vi "Cleanup Session.vi"(8 "error in":errorcluster, 11 "Plugin in":refnum<class "Output Sequencer.lvclass">) -> (0 "error out":errorcluster, 3 "Plugin out":refnum<class "Output Sequencer.lvclass">)   [LabVIEW 2024, in "Output Sequencer.lvlib" / "Output Sequencer.lvclass"]
uses:
  Output Sequencer.lvclass
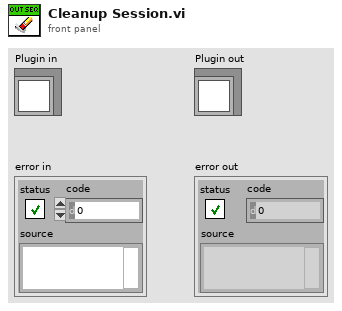
[diagram p1: front panel]
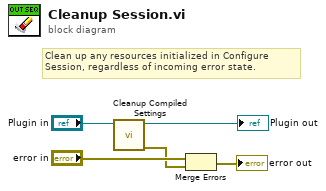
[diagram p0: block diagram]
diagram:
  # "Clean up any resources initialized in Configure Session, regardless of incoming error state."
  n1 = call "Cleanup Compiled Settings.vi"("Output Sequencer in"="Plugin in") -> ("error out"=w3:errorcluster, "Output Sequencer out"=→"Plugin out":refnum<class "Output Sequencer.lvclass">)  [unwired: 9 in]
  n2 = Merge Errors("error in", w3) -> (→"error out":errorcluster)
